vi "Enable Output.vi"(8 "error in (no error)":errorcluster, 10 "Output":bool, 11 "Agilent 33210A in":refnum<class "Agilent 33210A.lvclass">) -> (0 "error out":errorcluster, 3 "Agilent 33210A out":refnum<class "Agilent 33210A.lvclass">)   [LabVIEW 2016, in "Func Generator.lvlib" / "Agilent 33210A.lvclass"]
uses:
  Agilent 33210A.lvclass
  Agilent 33210A.lvclass/Agilent 33210A.ctl
  <instrlib>/Agilent 33XXX Series/Agilent 33XXX Series.lvlib
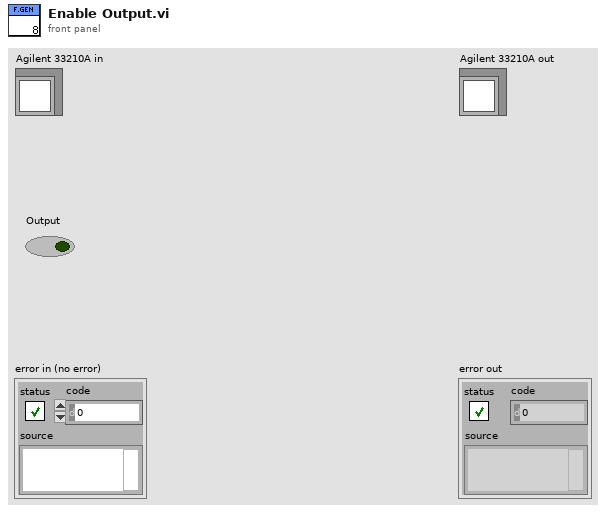
[diagram p1: front panel]
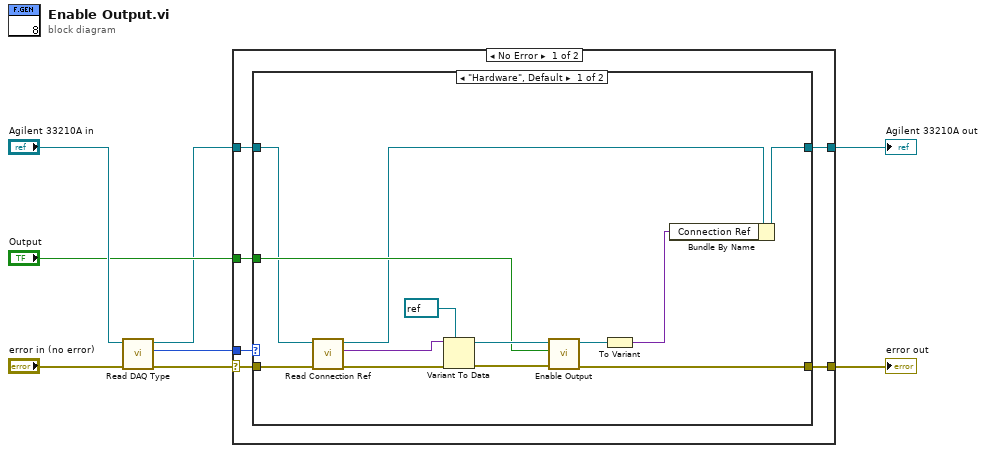
[diagram p0: block diagram]
diagram:
  n1 = call-dynamic "Read DAQ Type.vi"("error in (no error)"="error in (no error)", "Agilent 33210A in"="Agilent 33210A in") -> ("error out"=w7:errorcluster, "DAQ Type"=w6:enum16{"Hardware", "Simulation"}, "Agilent 33210A out"=w1:refnum<class "Agilent 33210A.lvclass">)  [unwired: 7 in]
  n2 = case shown="No Error" w7 {
    selector: w7 -> [w13 w30]
    tunnel: w6 -> [w14 _]
    tunnel: w1 -> [w12 w31]
    tunnel: "Output" -> [w11 _]
    tunnel: [w10 w31] -> w3
    tunnel: [w9 w30] -> w2
    frame No Error {
      n3 = case shown="\"Hardware\", Default" w14 {
        tunnel: w13 -> [w27 w28]
        tunnel: w12 -> [w16 w29]
        tunnel: w11 -> [w21 _]
        tunnel: [w20 w29] -> w10
        tunnel: [w18 w28] -> w9
        frame "Hardware", Default {
          n4 = call-dynamic "Read Connection Ref.vi"("error in (no error)"=w27, "Agilent 33210A in"=w16) -> ("error out"=w26:errorcluster, "Connection Ref"=w25:variant, "Agilent 33210A out"=w15:refnum<class "Agilent 33210A.lvclass">)  [unwired: 7 in]
          n5 = Variant To Data(error in=w26, type=refnum<visa-resource-name> refnum ("VISA resource name"), Variant=w25) -> (data=w22:refnum<visa-resource-name>, error out=w23:errorcluster)
          n6 = call <instrlib>:"Enable Output.vi"("error in (no error)"=w23, "Enable Output  (T: Enable)"=w21, "VISA resource name"=w22) -> ("error out"=w18:errorcluster, "VISA resource name out"=w19:refnum<visa-resource-name>)  [unwired: 7 in]
          n7 = To Variant(anything=w19) -> (Variant=w17:variant)
          n8 = Bundle By Name(cluster=w15, "Connection Ref"=w17) -> (w20:refnum<class "Agilent 33210A.lvclass">)
        }
        frame "Simulation" {
        }
      }
    }
    frame Error {
    }
  }
  "error out" <- w2
  "Agilent 33210A out" <- w3
